vi "HIOKI PW3390 Simple Acquisition.vi"() -> ()   [LabVIEW 2009]
doc: "Sets the output items except for the integration items and outputs the specified measurement data."
uses:
  <instrlib>/PW3390/Common/_Initialize/HIOKI PW3390 Initialize LAN.vi
  <instrlib>/PW3390/Common/_Initialize/HIOKI PW3390 Initialize RS-232C.vi
panel:
  out "error out":errorcluster
  in  "Communication Interface":enum16{"LAN", "RS-232C"}(ring)
  in  "COM Port":refnum<visa-resource-name>="COM1"
  in  "baud rate (38400bps)":u32=38400
  in  "IP Address":string="192.168.1.1"
  out "Data out":dbl[](array[numeric])
  out "Selected Item out":string[](array[string])
  in  "Option":T1
  in  "Efficiency":T2
  in  "I":T3
  in  "U":T3={"CH1"={"RMS"=TRUE, "MN "=FALSE, "AC  "=FALSE, "DC  "=FALSE, "FND"=FALSE, "THD"=FALSE, "PK+"=FALSE, "PK-"=FALSE}, "CH2"={"RMS"=TRUE, "MN "=FALSE, "AC  "=FALSE, "DC  "=FALSE, "FND"=FALSE, "THD"=FALSE, "PK+"=FALSE, "PK-"=FALSE}, "CH3"={"RMS"=TRUE, "MN "=FALSE, "AC  "=FALSE, "DC  "=FALSE, "FND"=FALSE, "THD"=FALSE, "PK+"=FALSE, "PK-"=FALSE}, "CH4"={"RMS"=TRUE, "MN "=FALSE, "AC  "=FALSE, "DC  "=FALSE, "FND"=FALSE, "THD"=FALSE, "PK+"=FALSE, "PK-"=FALSE}, "SUM12"={"RMS"=FALSE, "MN "=FALSE}, "SUM34"={"RMS"=FALSE, "MN "=FALSE}, "SUM123"={"RMS"=FALSE, "MN "=FALSE, "  -   "=FALSE, "UNB"=FALSE}}
  in  "Power Sum":T4
  in  "Power":T5
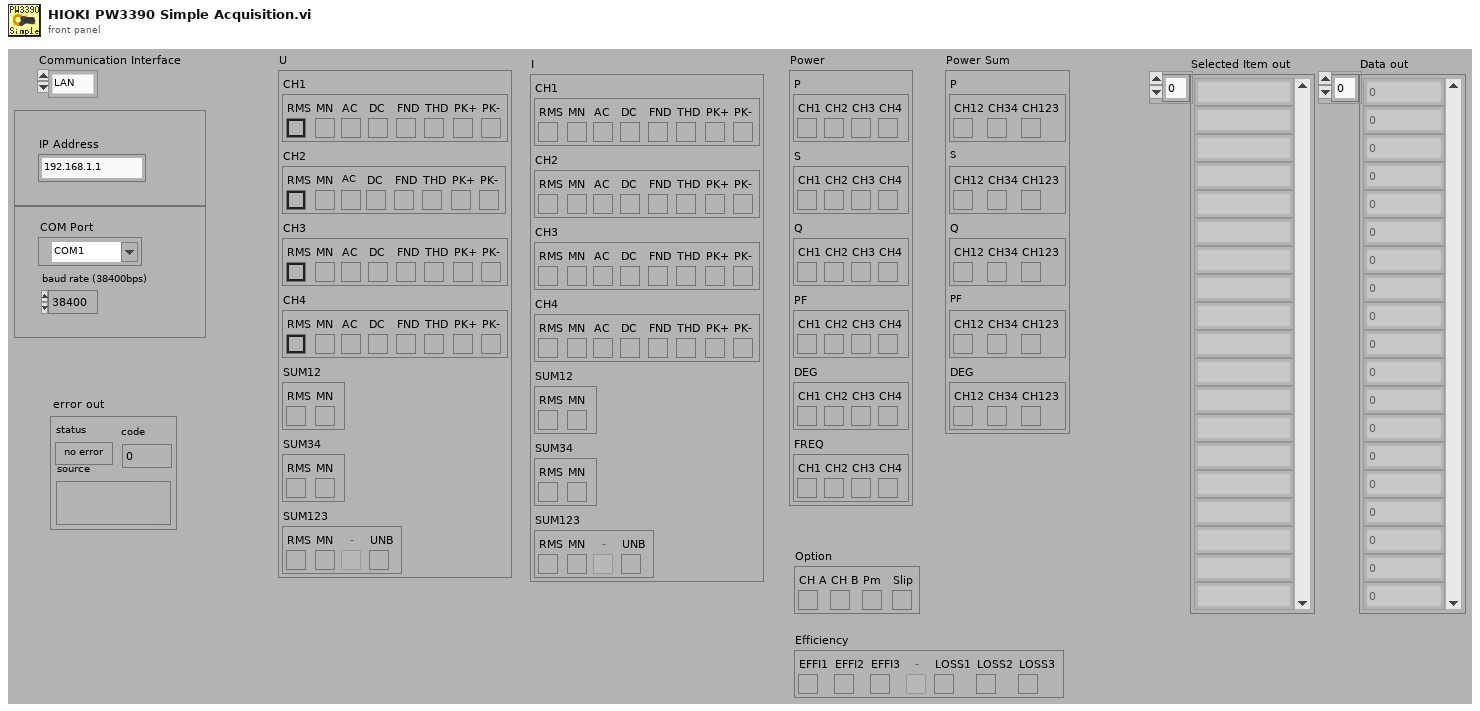
[diagram p1: front panel]
types:
  T1 = cluster{"CH A":bool, "CH B":bool, "Pm  ":bool, "Slip":bool}
  T2 = cluster{"EFFI1":bool, "EFFI2":bool, "EFFI3":bool, "  -   ":bool, "LOSS1":bool, "LOSS2":bool, "LOSS3":bool}
  T3 = cluster{"CH1":cluster{"RMS":bool, "MN ":bool, "AC  ":bool, "DC  ":bool, "FND":bool, "THD":bool, "PK+":bool, "PK-":bool}, "CH2":cluster{"RMS":bool, "MN ":bool, "AC  ":bool, "DC  ":bool, "FND":bool, "THD":bool, "PK+":bool, "PK-":bool}, "CH3":cluster{"RMS":bool, "MN ":bool, "AC  ":bool, "DC  ":bool, "FND":bool, "THD":bool, "PK+":bool, "PK-":bool}, "CH4":cluster{"RMS":bool, "MN ":bool, "AC  ":bool, "DC  ":bool, "FND":bool, "THD":bool, "PK+":bool, "PK-":bool}, "SUM12":cluster{"RMS":bool, "MN ":bool}, "SUM34":cluster{"RMS":bool, "MN ":bool}, "SUM123":cluster{"RMS":bool, "MN ":bool, "  -   ":bool, "UNB":bool}}
  T4 = cluster{"P":cluster{"CH12":bool, "CH34":bool, "CH123":bool}, "S":cluster{"CH12":bool, "CH34":bool, "CH123":bool}, "Q":cluster{"CH12":bool, "CH34":bool, "CH123":bool}, "PF":cluster{"CH12":bool, "CH34":bool, "CH123":bool}, "DEG":cluster{"CH12":bool, "CH34":bool, "CH123":bool}}
  T5 = cluster{"P":cluster{"CH1":bool, "CH2":bool, "CH3":bool, "CH4":bool}, "S":cluster{"CH1":bool, "CH2":bool, "CH3":bool, "CH4":bool}, "Q":cluster{"CH1":bool, "CH2":bool, "CH3":bool, "CH4":bool}, "PF":cluster{"CH1":bool, "CH2":bool, "CH3":bool, "CH4":bool}, "DEG":cluster{"CH1":bool, "CH2":bool, "CH3":bool, "CH4":bool}, "FREQ":cluster{"CH1":bool, "CH2":bool, "CH3":bool, "CH4":bool}}
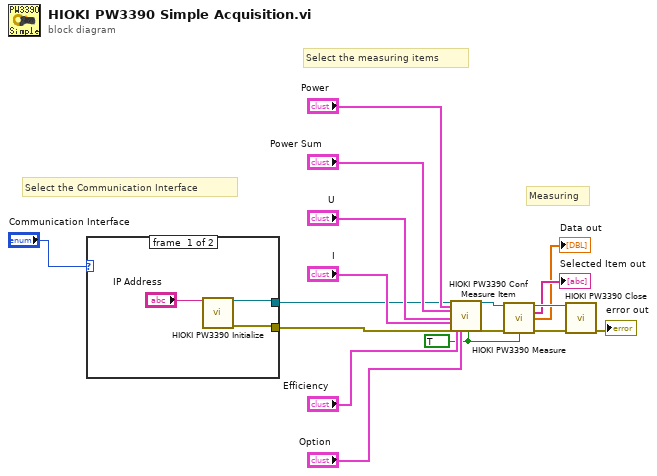
[diagram p0: block diagram]
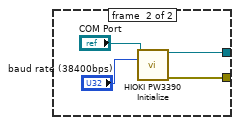
[diagram p2: hidden frame]
diagram:
  w1 = TRUE ("Error Out (F: Off)")
  # "Select the Communication Interface"
  # "Measuring"
  # "Select the measuring items"
  n1 = case shown="\"LAN\", デフォルト" "Communication Interface" {
    tunnel: [w19 w24] -> w4
    tunnel: [w18 w23] -> w3
    frame #0 {
      n2 = call-poly <instrlib>:"HIOKI PW3390 Initialize.vi"("IP Address"="IP Address") -> ("VISA Resource out"=w19:refnum<visa-resource-name>, "error out"=w18:errorcluster)  [unwired: 12 in, 1 out]
    }
    frame #1 {
      n3 = call-poly <instrlib>:"HIOKI PW3390 Initialize.vi"("COM Port"="COM Port", "baud rate (38400bps)"="baud rate (38400bps)") -> ("VISA Resource out"=w24:refnum<visa-resource-name>, "error out"=w23:errorcluster)  [unwired: 11 in, 1 out]
    }
  }
  n4 = call <instrlib>:"HIOKI PW3390 Conf Measure Item.vi"("VISA Resource"=w4, "Power"="Power", "Power Sum"="Power Sum", "U"="U", "I"="I", "error in (no error)"=w3, "Efficiency"="Efficiency", "Option"="Option", "Error Out (F: Off)"=w1) -> ("VISA Resource out"=w17:refnum<visa-resource-name>, "error out"=w15:errorcluster)  [unwired: 10 in, 7 out]
  n5 = call <instrlib>:"HIOKI PW3390 Measure.vi"("VISA Resource"=w17, "error in (no error)"=w15, "Error Out (F: Off)"=w1) -> ("VISA Resource out"=w16:refnum<visa-resource-name>, "Selected Item out"=→"Selected Item out":string[], "Data out"=→"Data out":dbl[], "error out"=w14:errorcluster)  [unwired: 7 in, 2 out]
  n6 = call <instrlib>:"HIOKI PW3390 Close.vi"("VISA Resource"=w16, "error in (no error)"=w14) -> ("error out"=→"error out":errorcluster)  [unwired: 13 in]
